vi "ProgressUpdate.vi"(7 "init":bool, 10 "add?":bool, 11 "DataBuffer":T1={"HMI"={"Download Progress"=refnum, "Status"=refnum, "SCU Info"=refnum, "PartType"=refnum}, "path"=path "", "CAN"={"Write Session in"="", "Read Session in"="", "TxRx Data"=[], "Response Good?"=FALSE, "spreadsheet string"="", "Rx Message"=[], "CAN frame"={"timestamp"=timestamp(0 s since 1904-01-01), "payload"=[2, 39, 3, 85, 85, 85, 85, 85], "identifier"=402391172, "type"=16, "extended?"=TRUE, "echo?"=FALSE}}, "error"={"status"=FALSE, "code"=0, "source"=""}, "CaseControl"={"histCase"=[], "retryCount"=0, "presentCase"=enum."Extend Session: 10 83", "nextEvent"=enum."Extend Session: 10 83"}, "NewEvent"={"Delay_ms"=0, "Case"=enum."Extend Session: 10 83", "Payload"=[], "Identifier"=0}, "Byte Log"=[], "Message"=refnum} {"CAN"."Tx CAN frame"."payload" format="%x"; "CAN"."Tx CAN frame"."timestamp" format="%<%.7X\n%x>T"; "CAN"."Tx CAN frame"."type" items=["CAN Data"=0, "CAN Remote"=1, "CAN Bus Error"=2, "CAN 2.0 Data"=8, "CAN FD Data"=16, "CAN FD+BRS Data"=24, "J1939 Data"=192, "Delay"=224, "Log Trigger"=225, "Start Trigger"=226]; "CAN"."Tx CAN frame"."identifier" format="%x"}) -> (2 "pass?":bool, 3 "DataBuffer":T1={"HMI"={"Download Progress"=refnum, "Status"=refnum, "SCU Info"=refnum, "PartType"=refnum}, "path"=path "", "CAN"={"Write Session in"="", "Read Session in"="", "TxRx Data"=[], "Response Good?"=FALSE, "spreadsheet string"="", "Rx Message"=[], "CAN frame"={"timestamp"=timestamp(0 s since 1904-01-01), "payload"=[2, 39, 3, 85, 85, 85, 85, 85], "identifier"=402391172, "type"=16, "extended?"=TRUE, "echo?"=FALSE}}, "error"={"status"=FALSE, "code"=0, "source"=""}, "CaseControl"={"histCase"=[], "retryCount"=0, "presentCase"=enum."Extend Session: 10 83", "nextEvent"=enum."Extend Session: 10 83"}, "NewEvent"={"Delay_ms"=0, "Case"=enum."Extend Session: 10 83", "Payload"=[], "Identifier"=0}, "Byte Log"=[], "Message"=refnum} {"CAN"."Tx CAN frame"."payload" format="%x"; "CAN"."Tx CAN frame"."timestamp" format="%<%.7X\n%x>T"; "CAN"."Tx CAN frame"."type" items=["CAN Data"=0, "CAN Remote"=1, "CAN Bus Error"=2, "CAN 2.0 Data"=8, "CAN FD Data"=16, "CAN FD+BRS Data"=24, "J1939 Data"=192, "Delay"=224, "Log Trigger"=225, "Start Trigger"=226]; "CAN"."Tx CAN frame"."identifier" format="%x"})   [LabVIEW 2018]
uses:
  Typedefs/DataBuffer.ctl
  <vilib>/xnet/xnet.llb/XNET Frame CAN.ctl
  <vilib>/xnet/xnet.llb/XNET Frame Type CAN.ctl
  TEST/Typedefs/Command.ctl
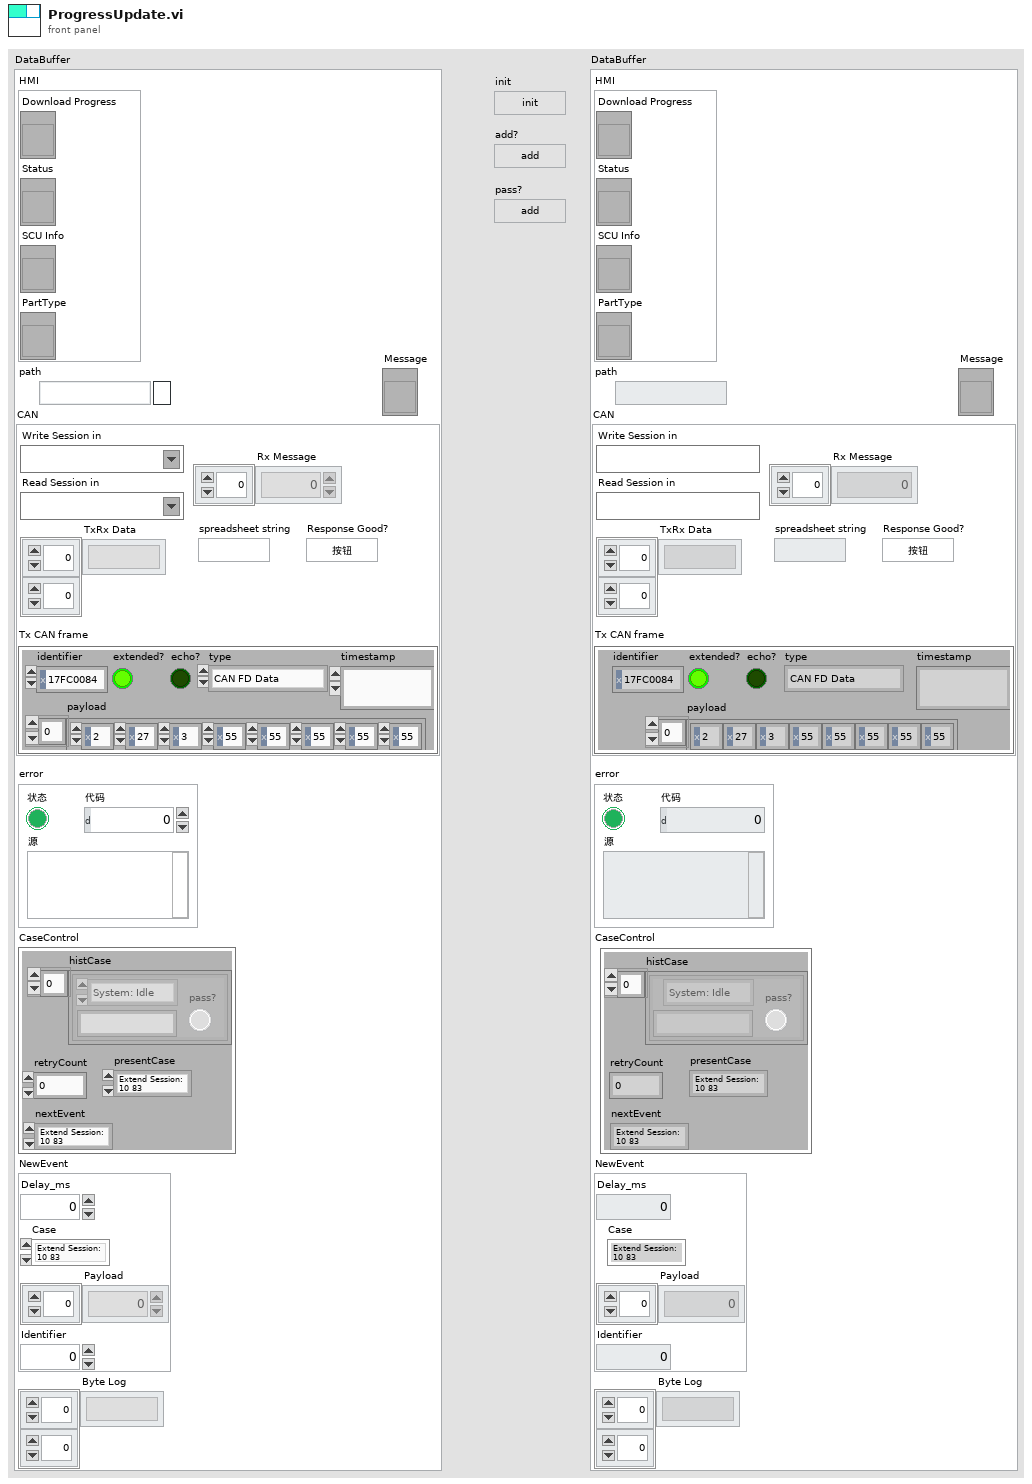
[diagram p1: front panel]
types:
  T1 = typedef "DataBuffer.ctl" = cluster{"HMI":cluster{"Download Progress":refnum<vi>, "Status":refnum<vi>, "SCU Info":refnum<vi>, "PartType":refnum<vi>}, "path":path, "CAN":cluster{"Write Session in":refnum<k21>, "Read Session in":refnum<k21>, "TxRx Data":string[][], "Response Good?":bool, "spreadsheet string":string, "Rx Message":u8[], "CAN frame":T2}, "error":errorcluster, "CaseControl":T4, "NewEvent":T6, "Byte Log":string[][], "Message":refnum<vi>}
  T2 = typedef "XNET Frame CAN.ctl" = cluster{"timestamp":timestamp, "payload":u8[], "identifier":u32, "type":T3, "extended?":bool, "echo?":bool}
  T3 = typedef "XNET Frame Type CAN.ctl" = u8
  T4 = typedef "CaseControl.ctl" = cluster{"histCase":cluster{"time":string, "event":T5, "pass?":bool}[], "retryCount":i32, "presentCase":T5, "nextEvent":T5}
  T5 = typedef "Command.ctl" = enum16{"Extend Session: 10 83", "Tester Present: 3E 80", "Resquest Seed: 27 01", "Send Key: 27 02", "Check FBL:  31 01 FD 02", "Control DTC: 85 82", "Comm Control: 28 83 01", "Program Session Request: 10 02", "Request Seed: 27 35", "Seed Key: 27 36", "Request Download: 34 00 44", "Transfer Data: 36 XX YY", "More Data?", "Request Transfer Exit: 37", "Check Flash Driver Validity: 01 FD 03", "More Segment?", "Write Data Fingereint: 23 F1 F0+26", "EraseFlashMemory Routine: 31 01 FD 00 44", "More segment?(each file)", "CheckAppSwAppData Validity: 31 01 FD 04 44", "CheckAppSwAppData Dependency: 31 01 fd 01", "ECU Reset: 11 81", "System: Init", "System: Idle", "System: Error", "System: Wait", "System: Delay", "System: CAN Send 1", "System: CAN Send 2", "System: CAN Read", "System: Exit"}
  T6 = typedef "NewEvent.ctl" = cluster{"Delay_ms":i32, "Case":T5, "Payload":u8[], "Identifier":u32}
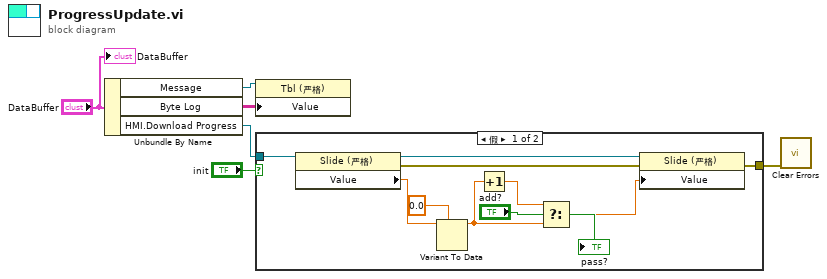
[diagram p0: block diagram]
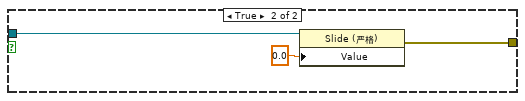
[diagram p2: hidden frame]
diagram:
  n1 = Unbundle By Name("DataBuffer") -> ("Message"=w2:refnum<vi>, "Byte Log"=w1:string[][], "HMI.Download Progress"=w6:refnum<vi>)
  n2 = property class="Tbl (严格)"(reference=w2, "Value"=w1) -> ()  [unwired: 1 in, 2 out]
  n3 = case shown="假" "init" {
    tunnel: w6 -> [w16 w19]
    tunnel: [w7 w17] -> w3
    frame False {
      n4 = property class="Slide (严格)"(reference=w16) -> (reference out=w13:refnum<vi>, error out=w8:errorcluster, "Value"=w15:dbl)  [unwired: 1 in]
      n5 = Variant To Data(type=0.0, Variant=w15) -> (data=w9:dbl)  [unwired: 1 in, 1 out]
      n6 = Increment(x=w9) -> (x+1=w10:dbl)
      n7 = Select(t=w10, s="add?", f=w9) -> (s? t:f=w11:dbl)
      n8 = property class="Slide (严格)"(reference=w13, error in=w8, "Value"=w11) -> (error out=w7:errorcluster)  [unwired: 1 out]
      "pass?" <- "add?"
    }
    frame True {
      n9 = property class="Slide (严格)"(reference=w19, "Value"=0.0) -> (error out=w17:errorcluster)  [unwired: 1 in, 1 out]
    }
  }
  n10 = call <vilib>:"Clear Errors.vi"("error in (no error)"=w3) -> ()  [unwired: 5 in, 2 out]
  "DataBuffer" <- "DataBuffer"
